vi "Error response to error cluster.vi"(7 "Status":string, 10 "error in (no error)":errorcluster, 11 "Response in":string) -> (2 "error out":errorcluster, 3 "Response out":string)   [LabVIEW 2019, in "CommandResponse communication.lvlib"]
uses:
  CommandResponse communication.lvlib
  Error response.ctl
  70d8b5ea-95d1-4cfa-ac5d-009d630f7c8c.vi
  70d8b5ea-95d1-4cfa-ac5d-009d630f7c8c.vi/efc1e533-85ae-4248-886a-f75999470694.vi
  70d8b5ea-95d1-4cfa-ac5d-009d630f7c8c.vi/04efa5ed-ca21-42a1-9699-91ac4a3dc900.vi
  <vilib>/Utility/High Resolution Relative Seconds.vi
  <vilib>/Utility/error.llb/Clear Errors.vi
  <vilib>/addons/_JKI.lib/Serialization/JSON/Library/Unflatten From JSON String.vi
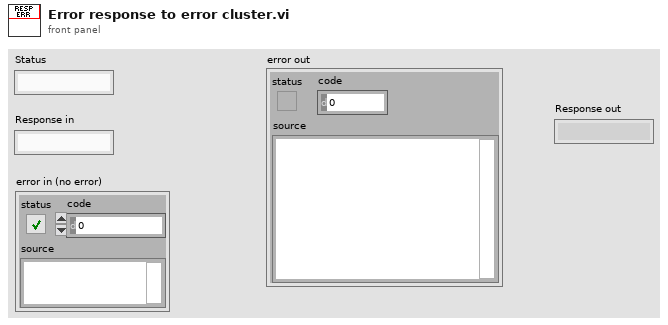
[diagram p1: front panel]
types:
  T1 = typedef "CommandResponse communication.lvlib/Error response.ctl" = cluster{"code":i32, "message":string, "source":string}
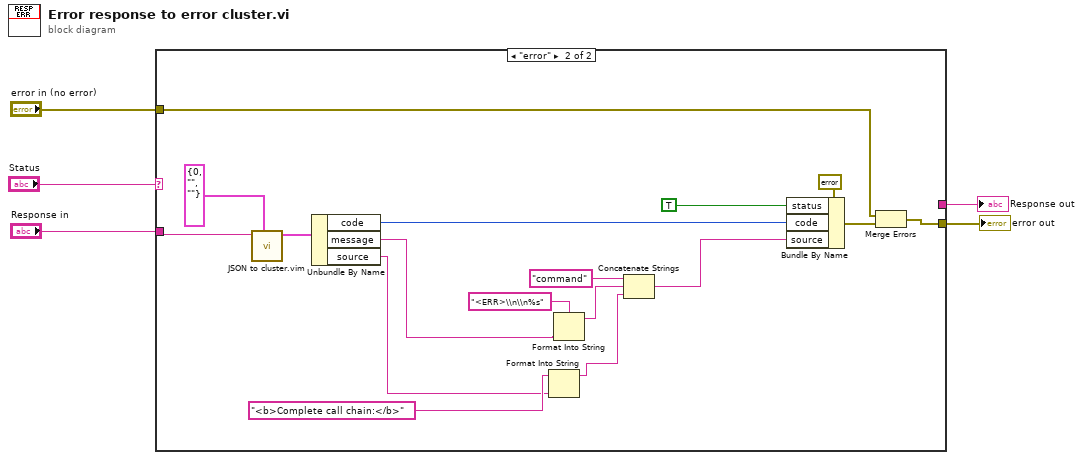
[diagram p0: block diagram]
diagram:
  n1 = case shown="\"error\"" "Status" {
    tunnel: [_ w14] -> w5
    tunnel: "Response in" -> [w6 w12]
    tunnel: [w6 _] -> w2
    tunnel: "error in (no error)" -> [_ w13]
    frame "OK", Default {
    }
    frame "error" {
      n2 = call "JSON to cluster.vim"("data"=T1 {"code"=0, "message"="", "source"=""} ("Error response"), "JSON in"=w12) -> ("data"=w10:T1)  [unwired: 7 in, 2 out]
      n3 = Unbundle By Name(w10) -> ("code"=w21:i32, "message"=w23:string, "source"=w8:string)
      n4 = Format Into String(initial string="<b>Complete call chain:</b>" ("regular expression"), w8) -> (resulting string=w7:string)  [unwired: 2 in, 1 out]
      n5 = Format Into String(format string="<ERR>\\n\\n%s" ("string"), w23) -> (resulting string=w16:string)  [unwired: 2 in, 1 out]
      n6 = Concatenate Strings("command" ("string"), w16, w7) -> (w19:string)
      n7 = Bundle By Name(cluster=errorcluster {"status"=FALSE, "code"=0, "source"=""} ("error constant"), "status"=TRUE, "code"=w21, "source"=w19) -> (w22:errorcluster)
      n8 = Merge Errors(w13, w22) -> (w14:errorcluster)
    }
  }
  "error out" <- w5
  "Response out" <- w2
